vi "Relative Pos to InterData Tunnel of CaseContent.vi"(8 "error in (no error)":errorcluster, 10 "element":string, 11 "CSM-Helper in":refnum<class "CSM-Helper.lvclass">) -> (0 "error out":errorcluster, 2 "Position":T1, 3 "CSM-Helper out":refnum<class "CSM-Helper.lvclass">)   [LabVIEW 2020, in "CSM-Helper.lvclass"]
uses:
  CSM-Helper.lvclass
  <vilib>/Utility/miscctls.llb/LVPositionTypeDef.ctl
  CSM-Helper.lvclass/CSM-Helper.ctl
  Properties/Read Case Structure Ref.vi
  API/Get CaseFrame Reference By CaseName.vi
  Properties/Read Front Tunnel Internal TermRefs.vi
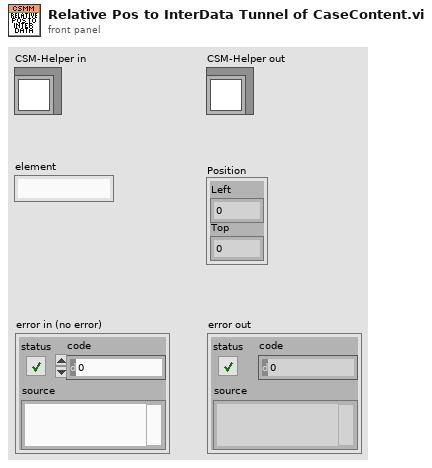
[diagram p1: front panel]
types:
  T1 = typedef "LVPositionTypeDef.ctl" = cluster{"Left":i32, "Top":i32}
  T2 = cluster{"InternalData":refnum<vi>, "CSM Name":refnum<vi>, "Last Resp":refnum<vi>, "Remaining State":refnum<vi>, "Arguments":refnum<vi>, "Response Source":refnum<vi>, "Source CSM":refnum<vi>, "Selector":refnum<vi>, "Error":refnum<vi>}
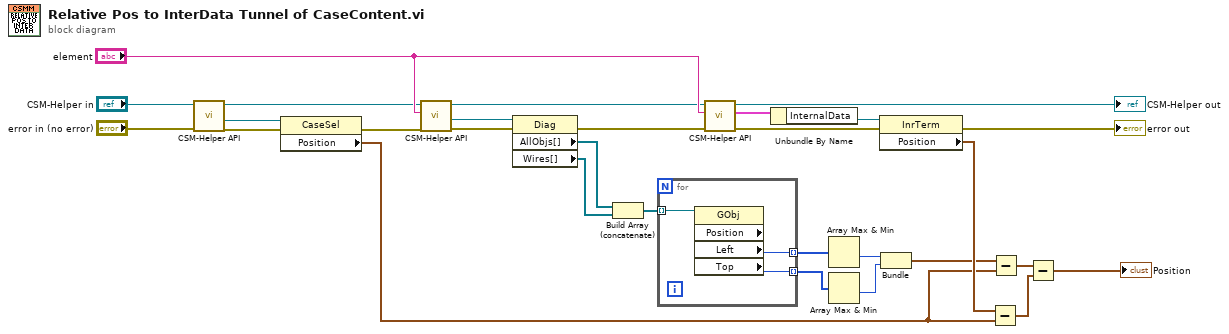
[diagram p0: block diagram]
diagram:
  n1 = call-poly "CSM-Helper API.vi"("error in (no error)"="error in (no error)", "CSM-Helper in"="CSM-Helper in") -> ("error out"=w22:errorcluster, "Case Structure"=w1:refnum<vi>, "CSM-Helper out"=w3:refnum<class "CSM-Helper.lvclass">)  [unwired: 7 in]
  n2 = property on="Property Node" class="CaseSel"(reference=w1, error in=w22) -> (error out=w23:errorcluster, "Position"=w16:T1)  [unwired: 1 out]
  n3 = call-poly "CSM-Helper API.vi"("error in (no error)"=w23, "CASE"="element", "CSM-Helper in"=w3) -> ("error out"=w25:errorcluster, "Frame Refs"=w2:refnum<vi>, "CSM-Helper out"=w12:refnum<class "CSM-Helper.lvclass">)  [unwired: 6 in]
  n4 = property on="Property Node" class="Diag"(reference=w2, error in=w25) -> (error out=w26:errorcluster, "AllObjs[]"=w6:refnum<vi>[], "Wires[]"=w7:refnum<vi>[])  [unwired: 1 out]
  n5 = Build Array (concatenate)(w6, w7) -> (w8:refnum<vi>[])
  n6 = for {
    tunnel: w8 -> [w32] mode=indexing
    tunnel: [w31] -> w5 mode=indexing
    tunnel: [w30] -> w4 mode=indexing
    n7 = property class="GObj" props=["Position", "Left", "Top"](reference=w32) -> ("Left"=w31:i32, "Top"=w30:i32)  [unwired: 1 in, 3 out]
  }
  n8 = call-poly "CSM-Helper API.vi"("error in (no error)"=w26, "case"="element", "CSM-Helper in"=w12) -> ("error out"=w24:errorcluster, "Front Tunnels"=w13:T2, "CSM-Helper out"=→"CSM-Helper out":refnum<class "CSM-Helper.lvclass">)  [unwired: 6 in]
  n9 = Unbundle By Name(w13) -> ("InternalData"=w14:refnum<vi>)
  n10 = Array Max & Min(array=w5) -> (min value=w9:i32)  [unwired: 3 out]
  n11 = Array Max & Min(array=w4) -> (min value=w10:i32)  [unwired: 3 out]
  n12 = property on="Property Node" class="InrTerm"(reference=w14, error in=w24) -> (error out=→"error out":errorcluster, "Position"=w17:T1)  [unwired: 1 out]
  n13 = Bundle(w9, w10) -> (w11:cluster{i32, i32})  [unwired: 1 in]
  n14 = Subtract(x=w17, y=w16) -> (x-y=w19:T1)
  n15 = Subtract(x=w11, y=w16) -> (x-y=w15:T1)
  n16 = Subtract(x=w15, y=w19) -> (x-y=→"Position":T1)
